vi "INHERITPUB.constructor.vi"(0 "name":string, 2 "data in":string, 5 "error in(no error)":errorcluster) -> (14 "i ref out":refnum<vi>, 16 "data out":string, 19 "error out":errorcluster)   [LabVIEW 2009]
doc: "This is the constructor of a class.\n\nLicense Agreement for this software:\n\nCopyright (C)\nGesellschaft für Schwerionenforschung, GSI\nPlanckstr. 1\n64291 Darmstadt\nGermany\n\nContact: D.Beck@gsi.de \n\nThis program is free software; you can redistribute it and/or modify it under the terms of the \nGNU General Public License as published by the Free Software Foundation; either version 2 of \nthe license, or (at your option) any later version.\n\nThis program is distributed in the hope that it will be useful, but WITHOUT ANY WARRANTY; \nwithout even the implied warranty of MERCHANTABILITY or FITNESS FOR A PARTICULAR PURPOSE. See the GNU General License for more details (http://www.gnu.org).\n\nGesellschaft für Schwerionenforschung, GSI\nPlanckstr. 1, 64291 Darmstadt, Germany\nFor all questions and ideas contact: M.Richter@gsi.de, H.Brand@gsi.de or D.Beck@gsi.de.\nLast update: 16-JUN-2004"
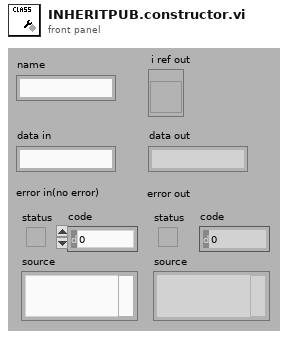
[diagram p1: front panel]
types:
  T1 = enum16{"SetAttribute", "GetAttribute", "CreateAttribute", "DestroyAttribute", "DestroyAllAtributes"}
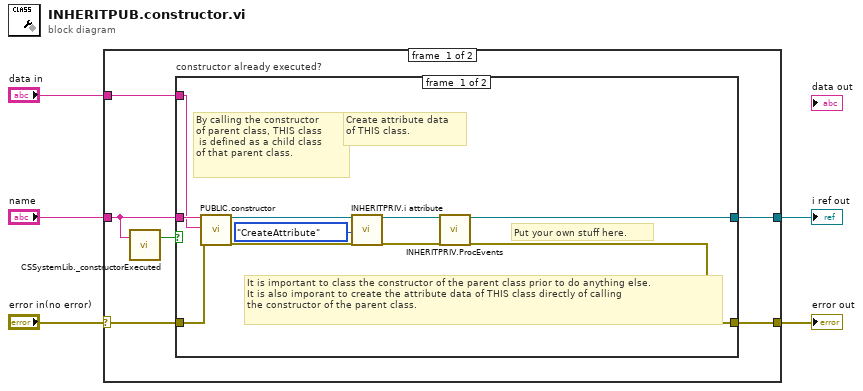
[diagram p0: block diagram]
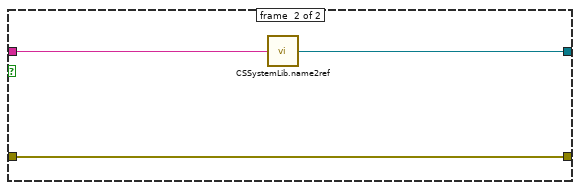
[diagram p2: hidden frame]
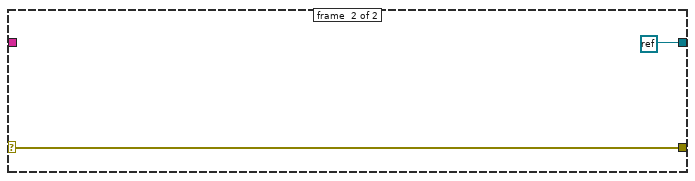
[diagram p3: hidden frame]
diagram:
  n1 = case shown="No Error" "error in(no error)" {
    selector: "error in(no error)" -> [w9 w25]
    tunnel: "name" -> [w8 _]
    tunnel: [w11 refnum<k0> refnum] -> w4
    tunnel: [w10 w25] -> w3
    tunnel: "data in" -> [w6 _]
    frame #0 {
      n2 = call "CSSystemLib._constructorExecuted.vi"("name"=w8) -> ("constructor executed?"=w7:bool)  [unwired: 18 in]
      n3 = case "constructor already executed?" shown="False" w7 {
        tunnel: w8 -> [w18 w24]
        tunnel: [w15 w23] -> w11
        tunnel: [w14 w22] -> w10
        tunnel: w9 -> [w13 w22]
        tunnel: w6 -> [w12 _]
        frame #0 {
          # "It is important to class the constructor of the parent class prior to do anything else.\nIt is also imporant to create the attribute data of THIS class directly of calling\nthe constructor of the parent class."
          # "Put your own stuff here."
          # "Create attribute data\nof THIS class."
          # "By calling the constructor\nof parent class, THIS class\n is defined as a child class\nof that parent class."
          n4 = call "PUBLIC.constructor.vi"("name"=w18, "data in"=w12, "error in(no error)"=w13) -> ("i ref out"=w21:refnum<vi>, "error out"=w20:errorcluster)  [unwired: 14 in, 1 out]
          n5 = call "INHERITPRIV.i attribute.vi"("VI Refnum"=w21, "Action"=T1."CreateAttribute", "error in (no error)"=w20) -> ("VI Refnum out"=w17:refnum<vi>, "error out"=w16:errorcluster)  [unwired: 14 in, 1 out]
          n6 = call "INHERITPRIV.ProcEvents.vi"("i ref in"=w17, "error in"=w16) -> ("i ref out"=w15:refnum<vi>, "error out"=w14:errorcluster)  [unwired: 16 in]
        }
        frame #1 {
          n7 = call "CSSystemLib.name2ref.vi"("name"=w24) -> ("obj refnum"=w23:refnum<vi>)
        }
      }
    }
    frame #1 {
    }
  }
  "i ref out" <- w4
  "error out" <- w3
